vi "Platinum - Convert mV to Kelvin.vi"(7 "Platinum mV":dbl format="%.4f") -> (8 "Platinum K":dbl format="%.4f")   [LabVIEW 2011]
panel:
  # "PLATINUM SENSOR"
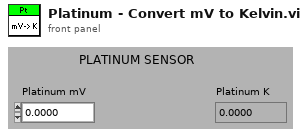
[diagram p1: front panel]
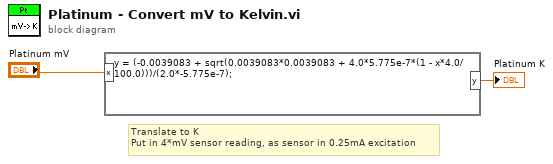
[diagram p0: block diagram]
diagram:
  # "Translate to K\nPut in 4*mV sensor reading, as sensor in 0.25mA excitation"
  n1 = formula code="y = (-0.0039083 + sqrt(0.0039083*0.0039083 + 4.0*5.775e-7*(1 - x*4.0/100.0)))/(2.0*-5.775e-7);"("x"="Platinum mV") -> ("y"=→"Platinum K":dbl)
